vi "gVar_ECa1.vi"() -> ()   [LabVIEW 2020]
panel:
  out "ECa1":dbl
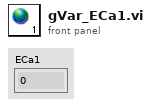
[diagram p1: front panel]
diagram:
